vi "factorial.vi"() -> ()   [LabVIEW 2018]
panel:
  out "Numeric 2":dbl
  in  "Numeric":i32
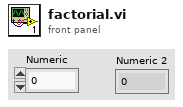
[diagram p1: front panel]
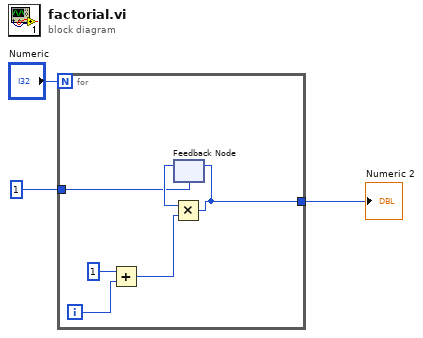
[diagram p0: block diagram]
diagram:
  n1 = for {
    N: "Numeric" -> [_]
    tunnel: 1 -> [w5]
    tunnel: [w4] -> w1
    i -> [w9]
    n2 = Add(x=1, y=w9) -> (x+y=w7:i32)
    n3 = feedback #1(w5) -> (w6:i32)
    n4 = Multiply(x=w6, y=w7) -> (x*y=w4:i32)
    n5 = feedback-in #1(w4) -> ()
  }
  "Numeric 2" <- w1
